vi "Turn Angle.vi"(8 "Tolerence":dbl=2.0 format="%#_13g", 9 "Process Variable type (Gyro)":enum16{"Gyro", "Vision target"}(ring), 10 "Motor Power":dbl=1.0, 11 "setpoint":dbl format="%.2f") -> (3 "In Range?":bool)   [LabVIEW 2015]
uses:
  Robot Values.vi
  <vilib>/addons/control/pid/NI_PID_pid.lvlib
  <vilib>/addons/control/pid/pid.llb/PID (DBL).vi
panel:
  out "In Range? (Old)":bool
  in  "output range":cluster{"output high":dbl, "output low":dbl}={"output high"=1.0, "output low"=-1.0} {"output low" format="%.2f"; "output high" format="%.2f"}
  in  "PID gains":T1={"proportional gain (Kc)"=0.010000000000000002, "integral time (Ti, min)"=0.0, "derivative time (Td, min)"=0.0} {"derivative time (Td, min)" format="%.3f"; "integral time (Ti, min)" format="%.3f"; "proportional gain (Kc)" format="%.3f"}
  # "Must be positive"
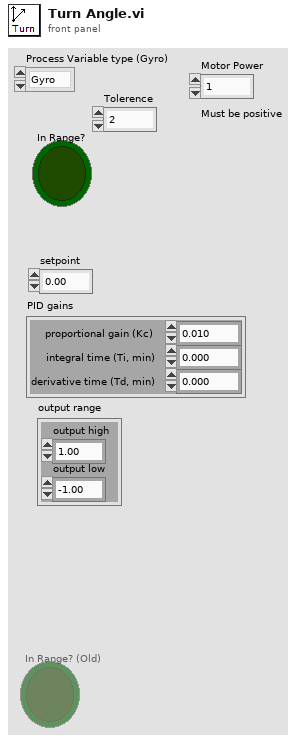
[diagram p1: front panel]
types:
  T1 = cluster{"proportional gain (Kc)":dbl, "integral time (Ti, min)":dbl, "derivative time (Td, min)":dbl}
  T2 = typedef "Robot Values.ctl" = cluster{"Drive Motors":cluster{"Left Motor Value":dbl, "Right Motor Value":dbl, "Left Motor Encoder":dbl, "Right Motor Encoder":dbl, "High/Low Gear":bool}, "Sensors":cluster{"Gyro Angle":dbl, "Photoeye":bool, "Ultrasonic Range":dbl, "Shooter Speed Encoder":dbl, "Accelerometer Value":dbl, "Flashlight":bool, "Target Distance":dbl, "Target X Value":dbl, "Reset Gyro?":bool}, "Arms":cluster{"Desired Arm Position":dbl, "Left Arm Encoder":dbl, "Right Arm Encoder":dbl, "Left Arm Lower Limit":bool, "Right Arm Lower Limit":bool, "Initialize Arm Position?":bool}, "Acquisition and Scoring":cluster{"Acquiring?":bool, "Current Speed":dbl, "Setpoint Speed":dbl, "Prep Wheels":bool, "Shoot":bool, "Low Eject":bool, "Reverse Shooter Wheel":bool}, "Hanging":cluster{"Pivot Arms":dbl, "PTO":bool, "Left Pivot Encoder":dbl, "Right Pivot Encoder":dbl, "Hanging Pin":bool}}
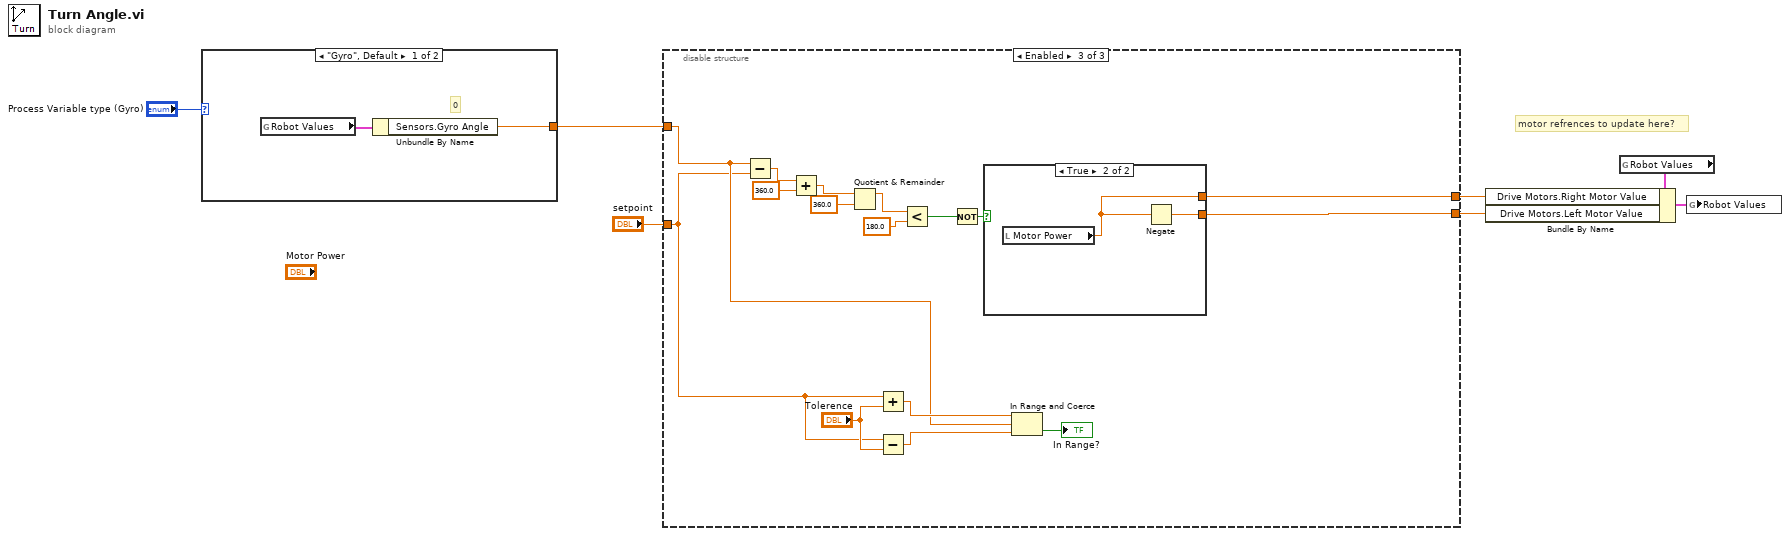
[diagram p0: block diagram]
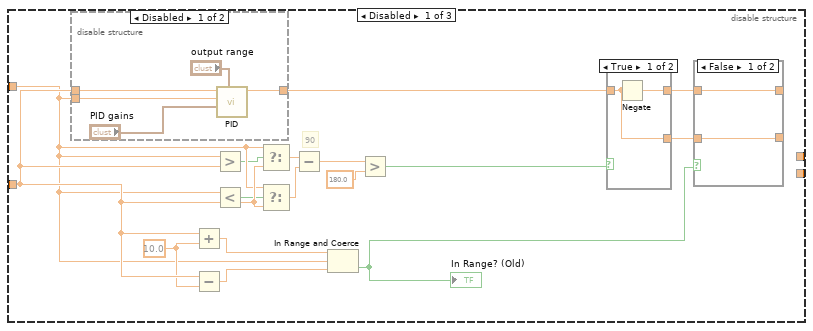
[diagram p2: hidden frame]
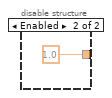
[diagram p3: hidden frame]
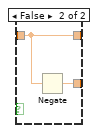
[diagram p5: hidden frame]
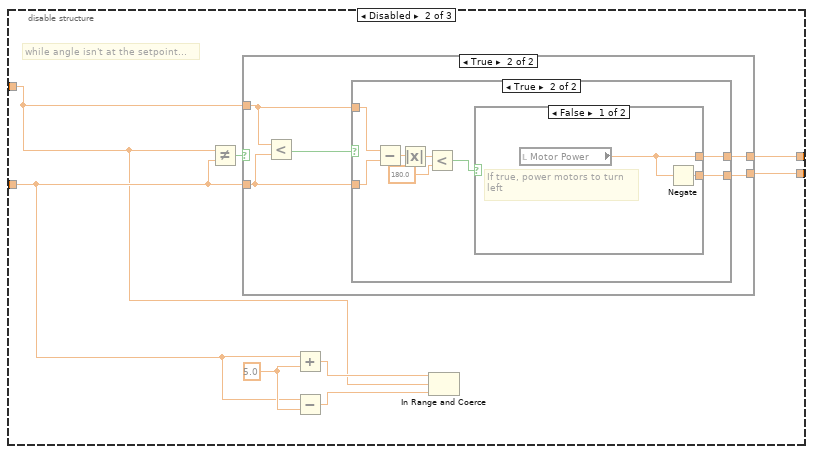
[diagram p6: hidden frame]
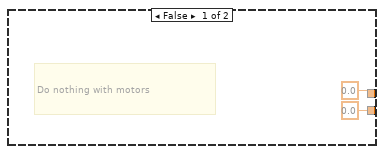
[diagram p7: hidden frame]
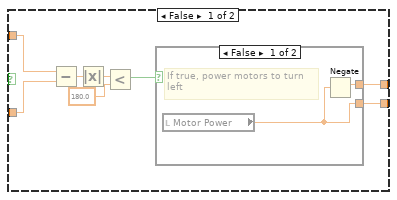
[diagram p8: hidden frame]
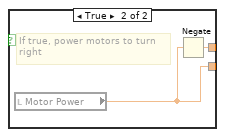
[diagram p9: hidden frame]
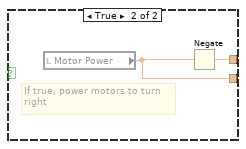
[diagram p10: hidden frame]
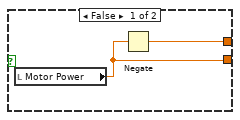
[diagram p11: hidden frame]
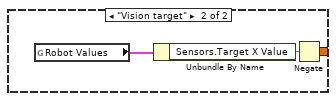
[diagram p12: hidden frame]
diagram:
  # "motor refrences to update here?"
  n1 = case shown="\"Gyro\", Default" "Process Variable type (Gyro)" {
    tunnel: [w8 w10] -> w3
    frame "Gyro", Default {
      # "0"
      n2 = global read "Robot Values.vi" "Robot Values"() -> (w9:T2)
      n3 = Unbundle By Name(w9) -> ("Sensors.Gyro Angle"=w8:dbl)
    }
    frame "Vision target" {
      n4 = global read "Robot Values.vi" "Robot Values"() -> (w12:T2)
      n5 = Unbundle By Name(w12) -> ("Sensors.Target X Value"=w11:dbl)
      n6 = Negate(x=w11) -> (-x=w10:dbl)
    }
  }
  n7 = disable-structure shown="Enabled" {
    disable-tunnel: "setpoint" -> [w28 w42 w83]
    disable-tunnel: w3 -> [w16 w41 w84]
    disable-tunnel: [_ w48 w88] -> w2
    disable-tunnel: [_ w47 w89] -> w1
    frame Disabled {
      w22 = 10.0
      # "90"
      n8 = disable-structure shown="Disabled" {
        disable-tunnel: w28 -> [w33 _]
        disable-tunnel: [w30 1.0] -> w23
        disable-tunnel: w16 -> [w29 _]
        frame Disabled {
          n9 = call-poly <vilib>:"PID.vi"("output range"="output range", "PID gains"="PID gains", "process variable"=w29, "setpoint"=w33) -> ("output"=w30:dbl)  [unwired: 6 in, 1 out]
        }
        frame Enabled {
        }
      }
      n10 = Add(x=w28, y=w22) -> (x+y=w21:dbl)
      n11 = Subtract(x=w28, y=w22) -> (x-y=w20:dbl)
      n12 = Greater?(x=w16, y=w28) -> (0:w15:bool)
      n13 = Less?(x=w16, y=w28) -> (x < y?=w14:bool)
      n14 = Select(t=w16, s=w15, f=w28) -> (s? t:f=w27:dbl)
      n15 = Select(t=w16, s=w14, f=w28) -> (s? t:f=w26:dbl)
      n16 = Subtract(x=w27, y=w26) -> (x-y=w13:dbl)
      n17 = In Range and Coerce(upper limit=w21, x=w16, lower limit=w20) -> (In Range?=w17:bool)  [unwired: 1 out]
      "In Range? (Old)" <- w17
      n18 = Greater?(x=w13, y=180.0) -> (0:w24:bool)
      n19 = case shown="True" w24 {
        tunnel: w23 -> [w38 w40]
        tunnel: [w37 w40] -> w19
        tunnel: [w38 w39] -> w18
        frame True {
          n20 = Negate(x=w38) -> (-x=w37:dbl)
        }
        frame False {
          n21 = Negate(x=w40) -> (-x=w39:dbl)
        }
      }
      n22 = case shown="False" w17 {
        tunnel: w19 -> [w36 _]
        tunnel: [w36 _] -> _
        tunnel: [w35 _] -> _
        tunnel: w18 -> [w35 _]
        frame False {
        }
        frame True {
        }
      }
    }
    frame Disabled {
      w46 = 5.0
      # "while angle isn't at the setpoint..."
      n23 = Not Equal?(x=w41, y=w42) -> (x != y?=w49:bool)
      n24 = case shown="True" w49 {
        tunnel: w41 -> [_ w55]
        tunnel: w42 -> [_ w54]
        tunnel: [0.0 w53] -> w48
        tunnel: [0.0 w52] -> w47
        frame False {
          # "Do nothing with motors"
        }
        frame True {
          n25 = Less?(x=w55, y=w54) -> (x < y?=w56:bool)
          n26 = case shown="True" w56 {
            tunnel: w55 -> [w64 w76]
            tunnel: w54 -> [w63 w75]
            tunnel: [w58 w70] -> w53
            tunnel: [w57 w69] -> w52
            frame False {
              n27 = Subtract(x=w64, y=w63) -> (x-y=w62:dbl)
              n28 = Absolute Value(x=w62) -> (abs(x)=w61:dbl)
              n29 = Less?(x=w61, y=180.0) -> (x < y?=w59:bool)
              n30 = case shown="False" w59 {
                tunnel: [w66 w68] -> w58
                tunnel: [w65 w67] -> w57
                frame False {
                  # "If true, power motors to turn\nleft"
                  n31 = local read "Motor Power"() -> (w66:dbl)
                  n32 = Negate(x=w66) -> (-x=w65:dbl)
                }
                frame True {
                  # "If true, power motors to turn\nright"
                  n33 = local read "Motor Power"() -> (w68:dbl)
                  n34 = Negate(x=w68) -> (-x=w67:dbl)
                }
              }
            }
            frame True {
              n35 = Subtract(x=w76, y=w75) -> (x-y=w74:dbl)
              n36 = Absolute Value(x=w74) -> (abs(x)=w73:dbl)
              n37 = Less?(x=w73, y=180.0) -> (x < y?=w71:bool)
              n38 = case shown="False" w71 {
                tunnel: [w77 w80] -> w70
                tunnel: [w78 w79] -> w69
                frame False {
                  # "If true, power motors to turn\nleft"
                  n39 = local read "Motor Power"() -> (w78:dbl)
                  n40 = Negate(x=w78) -> (-x=w77:dbl)
                }
                frame True {
                  # "If true, power motors to turn\nright"
                  n41 = local read "Motor Power"() -> (w80:dbl)
                  n42 = Negate(x=w80) -> (-x=w79:dbl)
                }
              }
            }
          }
        }
      }
      n43 = Add(x=w42, y=w46) -> (x+y=w45:dbl)
      n44 = Subtract(x=w42, y=w46) -> (x-y=w44:dbl)
      n45 = In Range and Coerce(upper limit=w45, x=w41, lower limit=w44) -> (In Range?=w43:bool)  [unwired: 1 out]
    }
    frame Enabled {
      n46 = Subtract(x=w84, y=w83) -> (x-y=w96:dbl)
      n47 = Add(x=w96, y=360.0) -> (x+y=w94:dbl)
      n48 = Quotient & Remainder(x=w94, y=360.0) -> (x-y*floor(x/y)=w92:dbl)  [unwired: 1 out]
      n49 = Add(x=w83, y="Tolerence") -> (x+y=w86:dbl)
      n50 = Subtract(x=w83, y="Tolerence") -> (x-y=w85:dbl)
      n51 = Less?(x=w92, y=180.0) -> (x < y?=w90:bool)
      n52 = Not(x=w90) -> (.not. x?=w81:bool)
      n53 = case shown="True" w81 {
        tunnel: [w97 w100] -> w89
        tunnel: [w98 w99] -> w88
        frame False {
          n54 = local read "Motor Power"() -> (w98:dbl)
          n55 = Negate(x=w98) -> (-x=w97:dbl)
        }
        frame True {
          n56 = local read "Motor Power"() -> (w100:dbl)
          n57 = Negate(x=w100) -> (-x=w99:dbl)
        }
      }
      n58 = In Range and Coerce(upper limit=w86, x=w84, lower limit=w85) -> (In Range?=→"In Range?":bool)  [unwired: 1 out]
    }
  }
  n59 = global read "Robot Values.vi" "Robot Values"() -> (w5:T2)
  n60 = Bundle By Name(cluster=w5, "Drive Motors.Right Motor Value"=w1, "Drive Motors.Left Motor Value"=w2) -> (w6:T2)
  n61 = global write "Robot Values.vi" "Robot Values"(w6) -> ()
